vi "Write to probe file.vi"() -> ()   [LabVIEW 2013]
uses:
  controls/Microprobe Vars.ctl
panel:
  in  "Microprobe state":T1 {"Gas C" format="%#_13g"; "Gas B" format="%#_13g"; "Gas A" format="%#_13g"; "Z" format="%#_13g"; "Y" format="%#_13g"; "X" format="%#_13g"; "Ramp rate" format="%#_13g"; "Telem" format="%#_13g"}
  out "error out":errorcluster
  out "path":path
  in  "error in":errorcluster
  in  "Sample name":string
  in  "Directory":path
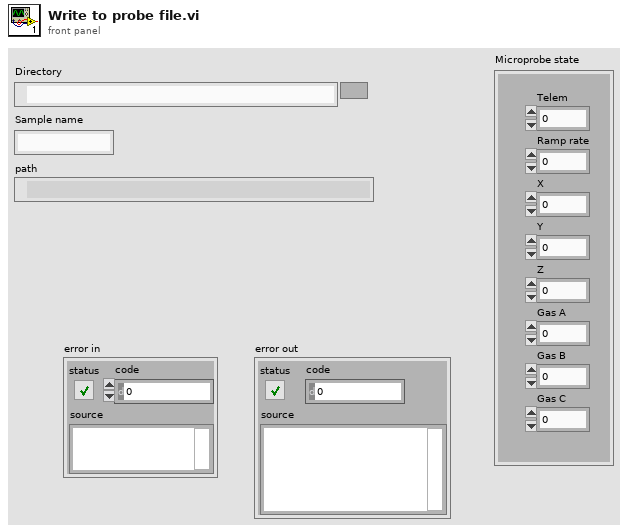
[diagram p1: front panel]
types:
  T1 = typedef "Microprobe Vars.ctl" = cluster{"Telem":dbl, "Ramp rate":dbl, "X":dbl, "Y":dbl, "Z":dbl, "Gas A":dbl, "Gas B":dbl, "Gas C":dbl}
  T2 = enum16{"open", "replace", "create", "open or create", "replace or create", "replace or create with confirmation"}
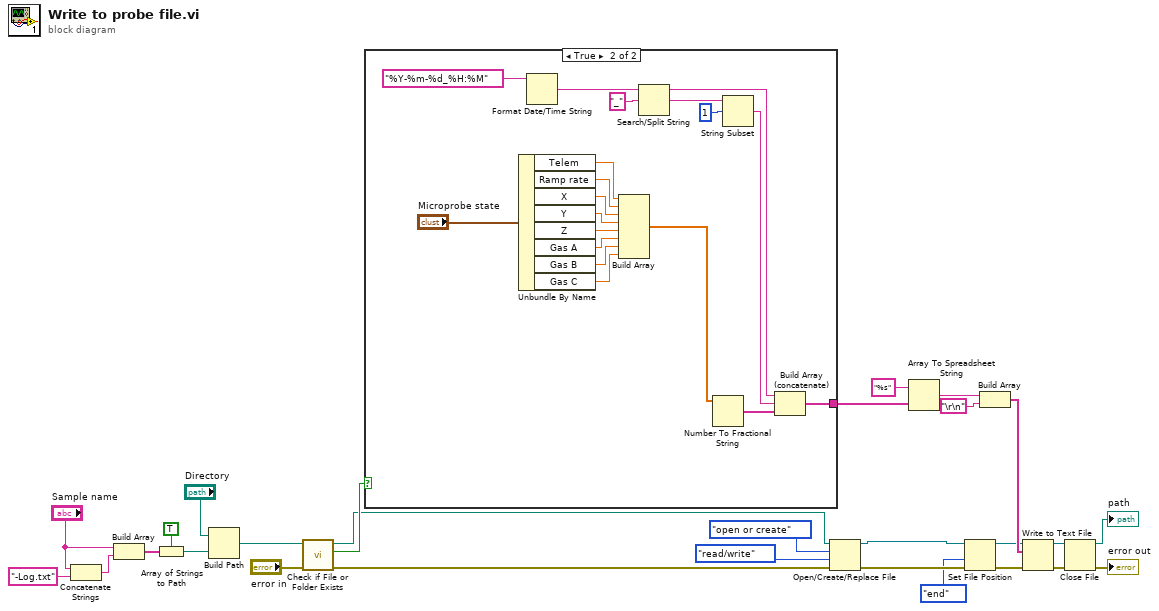
[diagram p0: block diagram]
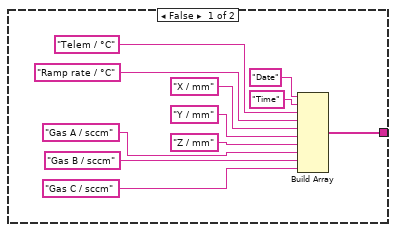
[diagram p2: hidden frame]
diagram:
  n1 = Concatenate Strings("Sample name", "-Log.txt" ("string")) -> (w23:string)
  n2 = Build Array("Sample name", w23) -> (w27:string[])
  n3 = Array of Strings to Path(0:w27, 1:TRUE ("relative")) -> (2:w22:path)
  n4 = Build Path(base path="Directory", name or relative path=w22) -> (appended path=w15:path)
  n5 = call <vilib>:"Check if File or Folder Exists.vi"("error in (no error)"="error in", "path"=w15) -> ("error out"=w13:errorcluster, "file or folder exists?"=w25:bool, "dup path"=w16:path)  [unwired: 7 in]
  n6 = case shown="True" w25 {
    tunnel: [w29 w51] -> w18
    frame False {
      n7 = Build Array("Date", "Time", "Telem / °C", "Ramp rate / °C", "X / mm", "Y / mm", "Z / mm", "Gas A / sccm", "Gas B / sccm", "Gas C / sccm") -> (w29:string[])
    }
    frame True {
      n8 = Unbundle By Name("Microprobe state") -> ("Telem"=w47:dbl, "Ramp rate"=w46:dbl, "X"=w45:dbl, "Y"=w44:dbl, "Z"=w43:dbl, "Gas A"=w42:dbl, "Gas B"=w41:dbl, "Gas C"=w40:dbl)
      n9 = Format Date/Time String(time format string (%c)="%Y-%m-%d_%H:%M") -> (date/time string=w57:string)  [unwired: 2 in]
      n10 = Build Array(w47, w46, w45, w44, w43, w42, w41, w40) -> (w50:dbl[])
      n11 = Search/Split String(string=w57, search string/char (-)="_") -> (substring before match=w52:string, match + rest of string=w55:string)  [unwired: 1 in, 1 out]
      n12 = Number To Fractional String(number=w50) -> (F-format string=w49:string[])  [unwired: 3 in]
      n13 = String Subset(string=w55, offset (0)=1) -> (substring=w53:string)  [unwired: 1 in]
      n14 = Build Array (concatenate)(w52, w53, w49) -> (w51:string[])
    }
  }
  n15 = Open/Create/Replace File(file path (use dialog)=w16, error in=w13, operation (0:open)=T2."open or create", access (0:read/write)=enum16{"read/write", "read-only", "write-only"}."read/write") -> (refnum out=w8:refnum<file>, error out=w7:errorcluster)  [unwired: 2 in, 1 out]
  n16 = Array To Spreadsheet String(array=w18, 3:"%s" ("format string")) -> (spreadsheet string=w5:string)  [unwired: 1 in]
  n17 = Set File Position(refnum=w8, from (0:start)=enum16{"start", "end", "current"}."end", error in=w7) -> (refnum out=w2:refnum<file>, error out=w1:errorcluster)  [unwired: 1 in]
  n18 = Build Array(w5, "\r\n") -> (w3:string[])
  n19 = Write to Text File(file (use dialog)=w2, text=w3, error in=w1) -> (refnum out=w12:refnum<file>, error out=w11:errorcluster)  [unwired: 1 in, 1 out]
  n20 = Close File(refnum=w12, error in=w11) -> (path=→"path":path, error out=→"error out":errorcluster)
